vi "Reset Supply.vi"(8 "error in":errorcluster, 11 "89XX in":refnum<class "89XX.lvclass">) -> (0 "error out":errorcluster, 3 "89XX out":refnum<class "89XX.lvclass">)   [LabVIEW 2019, in "89XX.lvlib" / "89XX.lvclass"]
uses:
  Library/89XX.lvclass
  Library/89XX.lvclass/89XX.ctl
  builds/Instruments/PowerSupply.lvlibp/Library/PowerSupply.lvclass
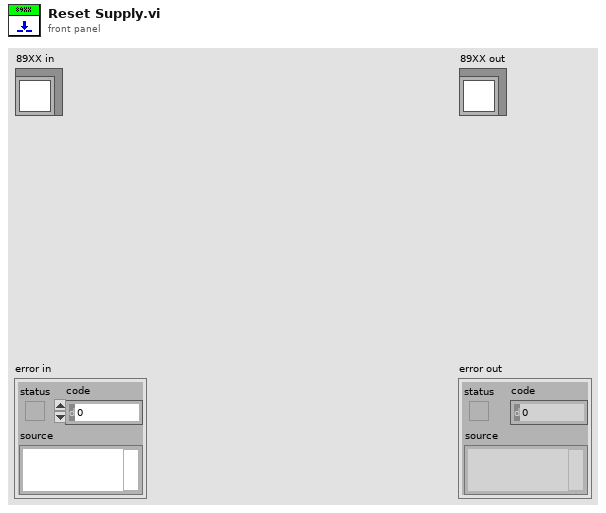
[diagram p1: front panel]
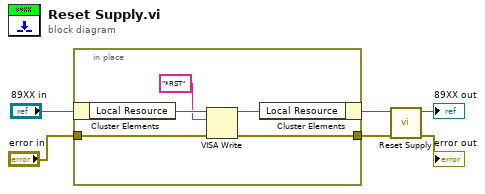
[diagram p0: block diagram]
diagram:
  n1 = in-place {
    in-place-border: [w9] -> w3
    in-place-border: "error in" -> [w7]
    n2 = in-place-cluster #1("89XX in") -> ("Local Resource"=w11:refnum<visa-resource-name>)
    n3 = VISA Write(VISA resource name=w11, write buffer="*RST", error in (no error)=w7) -> (VISA resource name out=w10:refnum<visa-resource-name>, error out=w9:errorcluster)  [unwired: 1 out]
    n4 = in-place-cluster #1("Local Resource"=w10) -> (w1:refnum<class "89XX.lvclass">)
  }
  n5 = call-parent "Reset Supply.vi"("error in"=w3, "PowerSupply in"=w1) -> ("error out"=→"error out":errorcluster, "PowerSupply out"=→"89XX out":refnum<class "89XX.lvclass">)  [unwired: 8 in]
